vi "getUnit.vi"(8 "error in (no error)":errorcluster, 11 "Electrometer in":refnum<class "Electrometer.lvclass">) -> (0 "error out":errorcluster, 2 "Unit":string, 3 "Electrometer out":refnum<class "Electrometer.lvclass">)   [LabVIEW 2016, in "Electrometer.lvclass"]
uses:
  Electrometer.lvclass
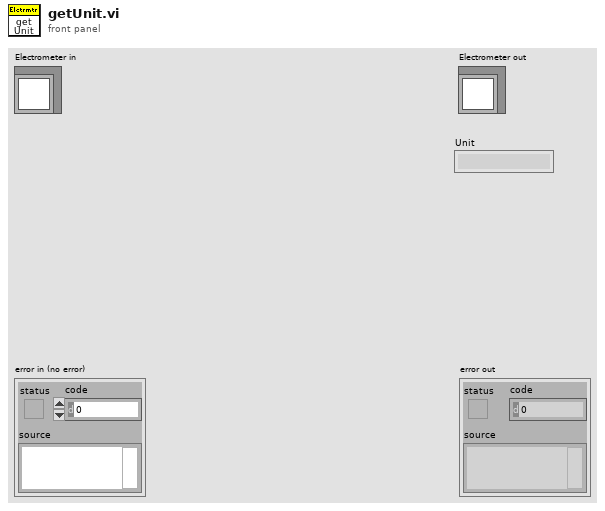
[diagram p1: front panel]
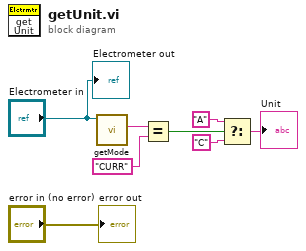
[diagram p0: block diagram]
diagram:
  n1 = call "getMode.vi"("Electrometer in"="Electrometer in") -> ("Mode"=w2:string)  [unwired: 8 in, 2 out]
  n2 = Equal?(x=w2, y="CURR") -> (x = y?=w6:bool)
  n3 = Select(t="A", s=w6, f="C") -> (s? t:f=→"Unit":string)
  "error out" <- "error in (no error)"
  "Electrometer out" <- "Electrometer in"
